vi "1-Palindromic Word Detector.vi"() -> ()   [LabVIEW 2014]
panel:
  out "Reverse":string
  out "Lower Case":string
  out "Boolean":bool
  in  "Word":string
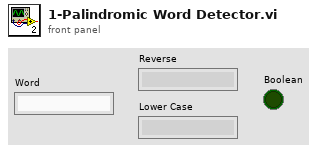
[diagram p1: front panel]
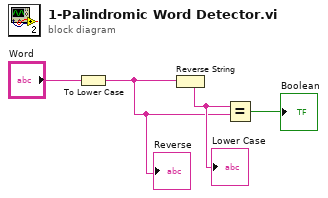
[diagram p0: block diagram]
diagram:
  n1 = To Lower Case(string="Word") -> (all lower case string=w1:string)
  "Reverse" <- w1
  n2 = Reverse String(1:w1) -> (0:w2:string)
  "Lower Case" <- w2
  n3 = Equal?(x=w2, y=w1) -> (x = y?=→"Boolean":bool)
